vi "libssh2_session_handshake.vi"   [LabVIEW 2017, in "libssh2.lvlib"]
doc: "Perform the SSH handshake on a session.\n\nAfter handshake, verify the remote host key using libssh2_session_hostkey and libssh2_knownhost_checkp before any authentication."
uses:
  libssh2.lvlib
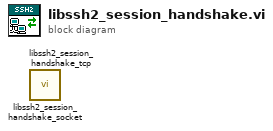
[diagram p0: block diagram]
diagram:
  n1 = call "libssh2_session_handshake_socket.vi"() -> ()  [unwired: 11 in, 1 out]
  n2 = call "libssh2_session_handshake_tcp.vi"() -> ()  [unwired: 11 in, 1 out]
